vi "Control commands to FPGA.vi"(0 "FPGA Interface":refnum<k20>, 1 "error in (no error)":errorcluster, 2 "LQR direction":bool, 3 "Duty cycle (Only used for LQR)":dbl, 4 "Controller output":dbl, 6 "Reset steering angle":bool, 8 "Reset steering\nposition controller":bool) -> (14 "FPGA VI Reference Out":refnum<k20>, 15 "error out":errorcluster, 19 "Log?":dbl)   [LabVIEW 2016]
uses:
  <vilib>/Utility/error.llb/Error Cluster From Error Code.vi
  <vilib>/rvi/errors/niLvFpgaAdjustHostInterfaceError.vi
  <vilib>/rvi/interface/nirviReadWriteControl/nirviReadWriteControl.xnode
  <vilib>/rvi/interface/nirviMethod/nirviMethod.xnode
  NiFpgaLv.dll
  <vilib>/rvi/interface/Simulation/niFpgaSimulationCallBeginRW.vi
  <vilib>/FPGAPlugInAG/Dynamic/niLvFpga_WriteFifo_Dynamic.vi
  <vilib>/rvi/errors/niLvFpgaMergeErrorWithErrorCode.vi
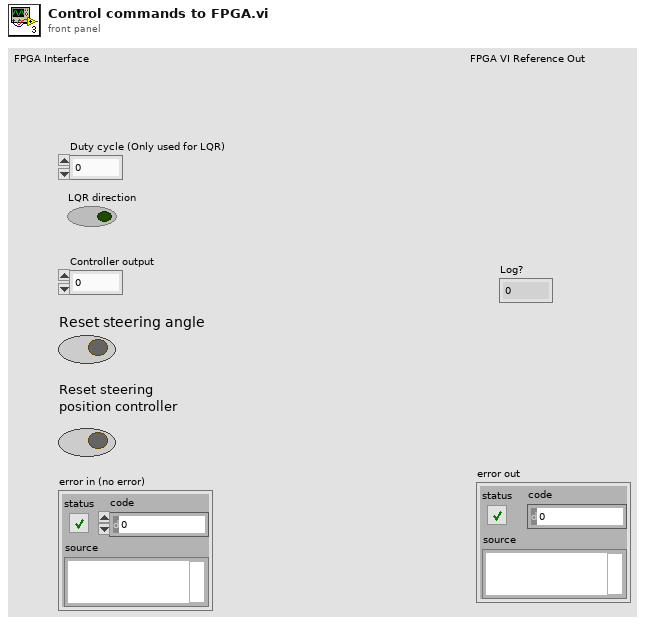
[diagram p1: front panel]
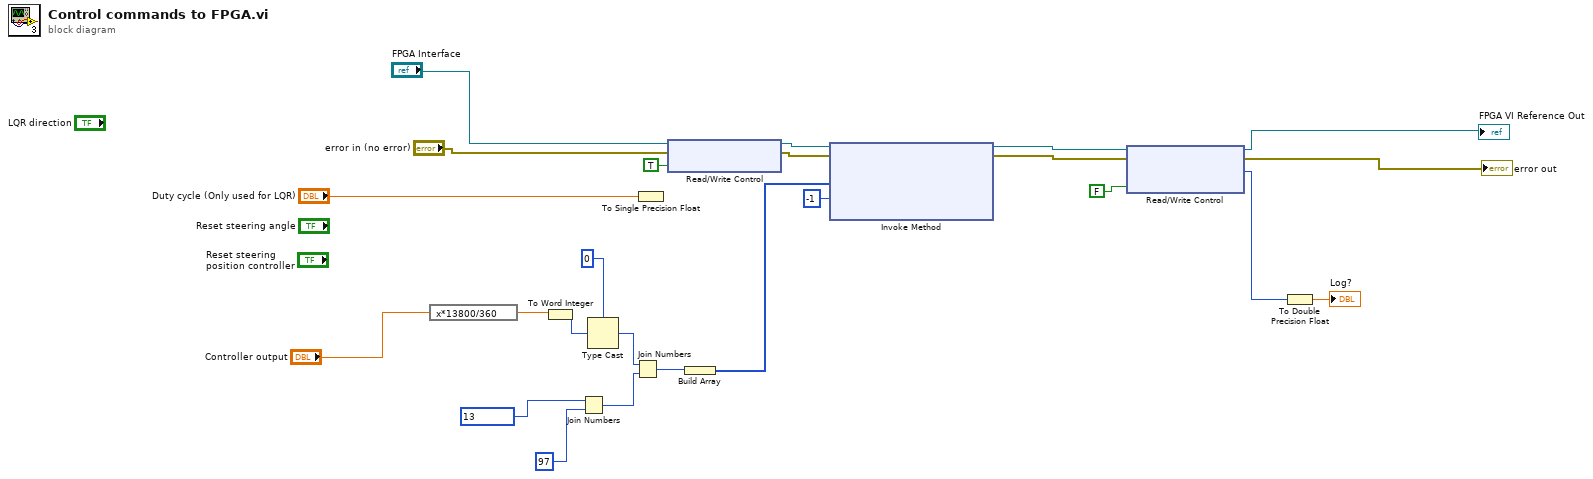
[diagram p0: block diagram]
diagram:
  n1 = expression code="x*13800/360"("Controller output") -> (w2:dbl)
  n2 = To Word Integer(number=w2) -> (16bit integer=w9:i16)
  n3 = Join Numbers(hi=u8 13, lo=u8 97) -> ((hi.lo)=w12:u16)
  n4 = Type Cast(type=u16 0, x=w9) -> (*(type *) &x=w7:u16)
  n5 = Join Numbers(hi=w7, lo=w12) -> ((hi.lo)=w6:u32)
  n6 = To Single Precision Float(number="Duty cycle (Only used for LQR)") -> ()  [unwired: 1 out]
  n7 = xnode "Read/Write Control"("FPGA VI Reference In"="FPGA Interface", "error in"="error in (no error)", "ODrive RT Control"=TRUE) -> ("FPGA VI Reference Out"=w17:refnum<k20>, "error out"=w18:errorcluster)
  n8 = Build Array(w6) -> (w5:u32[])
  n9 = xnode "Invoke Method"("FPGA VI Reference In"=w17, "error in"=w18, "Data"=w5, "Timeout (ms)"=-1) -> ("FPGA VI Reference Out"=w15:refnum<k20>, "error out"=w16:errorcluster)  [unwired: 1 out]
  n10 = xnode "Read/Write Control"("FPGA VI Reference In"=w15, "error in"=w16, "ODrive RT Control"=FALSE) -> ("FPGA VI Reference Out"=→"FPGA VI Reference Out":refnum<k20>, "error out"=→"error out":errorcluster, "Channel 7 position"=w22:u8)
  n11 = To Double Precision Float(number=w22) -> (double precision float=→"Log?":dbl)
